vi "Add VIs and their Protperties to Tree.vi"(5 "Globals?":bool, 6 "File Extension Filters":string[](array[string]), 7 "Exclude vi.lib?":bool, 8 "error in":errorcluster, 10 "AppInst":refnum<vi>, 11 "Data Tree":refnum<vi>) -> (0 "error out":errorcluster)   [LabVIEW 2009]
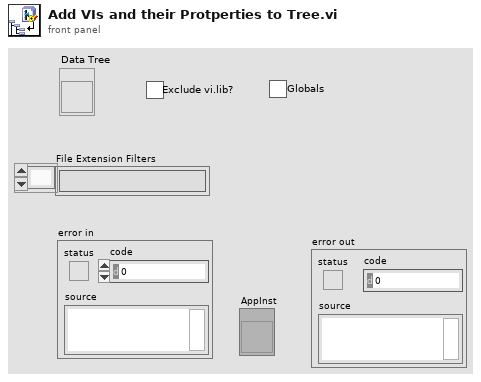
[diagram p1: front panel]
types:
  T1 = enum32{"invalid VI type", "Standard VI", "Control VI", "Global VI", "Polymorphic VI", "Configuration VI", "SubSystem", "Facade VI", "Method VI", "Statechart Diagram VI"}
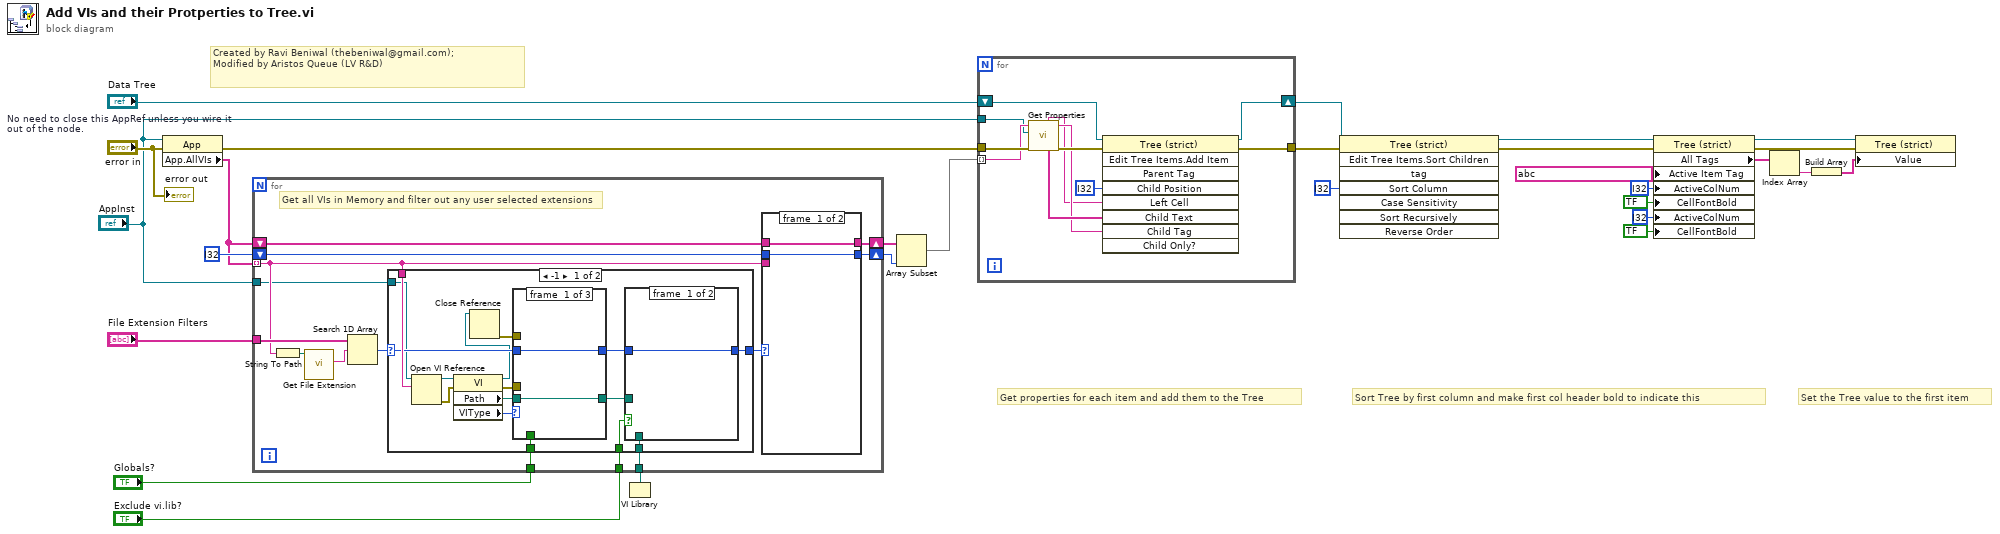
[diagram p0: block diagram]
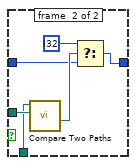
[diagram p2: hidden frame]
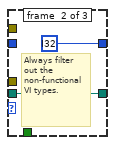
[diagram p3: hidden frame]
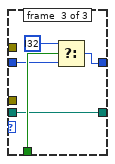
[diagram p4: hidden frame]
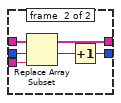
[diagram p6: hidden frame]
diagram:
  # "Sort Tree by first column and make first col header bold to indicate this"
  # "Created by Ravi Beniwal (thebeniwal@gmail.com);\nModified by Aristos Queue (LV R&D)"
  # "Set the Tree value to the first item"
  # "Get properties for each item and add them to the Tree"
  n1 = property on="No need to close this AppRef unless you wire it out of the node." class="App"(reference="AppInst", error in="error in") -> (error out=w5:errorcluster, "App.AllVIs"=w22:string[])  [unwired: 1 out]
  n2 = VI Library() -> (path=w2:path)
  n3 = for {
    tunnel: w22 -> [w33] mode=indexing
    tunnel: "File Extension Filters" -> [w41]
    shift-right: [w38] -> w24
    shift-left: w22 -> [w39]
    shift-right: [w36] -> w23
    shift-left: i32 ? -> [w37]
    tunnel: "Globals?" -> [w32]
    tunnel: "Exclude vi.lib?" -> [w31]
    tunnel: w2 -> [w30]
    tunnel: "AppInst" -> [w29]
    # "Get all VIs in Memory and filter out any user selected extensions"
    n4 = String To Path(string=w33) -> (path=w42:path)
    n5 = call <vilib>:"Get File Extension.vi"("file"=w42) -> ("lowercase file extension"=w40:string)  [unwired: 7 in, 3 out]
    n6 = Search 1D Array(1D array=w41, element=w40) -> (index of element=w35:i32)  [unwired: 1 in]
    n7 = case shown="-1" w35 {
      selector: w35 -> [w55 w75]
      tunnel: [w48 w75] -> w34
      tunnel: w33 -> [w58 _]
      tunnel: w32 -> [w53 _]
      tunnel: w31 -> [w52 _]
      tunnel: w30 -> [w50 _]
      tunnel: w29 -> [w43 _]
      frame #0 {
        n8 = Open VI Reference(application reference (local)=w43, vi path=w58) -> (vi reference=w57:refnum<vi>, error out=w46:errorcluster)  [unwired: 4 in]
        n9 = property class="VI"(reference=w57, error in=w46) -> (reference out=w47:refnum<vi>, error out=w45:errorcluster, "Path"=w54:path, "VIType"=w56:T1)
        n10 = Close Reference(reference=w47) -> (error out=w44:errorcluster)  [unwired: 1 in]
        n11 = case shown="\"Polymorphic VI\", \"Configuration VI\"" w56 {
          tunnel: w55 -> [w67 _ w73]
          tunnel: [w67 i32 ? ("index of element") w72] -> w49
          tunnel: w54 -> [w66 w68 w70]
          tunnel: w53 -> [_ _ w74]
          tunnel: [w66 w68 w70] -> w51
          tunnel: w45 -> [_ _ _]
          tunnel: w44 -> [_ _ _]
          frame #0 {
          }
          frame #1 {
            # "Always filter out the non-functional VI types."
          }
          frame #2 {
            n12 = Select(t=i32 ?, s=w74, f=w73) -> (s? t:f=w72:i32)
          }
        }
        n13 = case shown="True" w52 {
          tunnel: w51 -> [_ w65]
          tunnel: w50 -> [_ w64]
          tunnel: w49 -> [w59 w62]
          tunnel: [w59 w60] -> w48
          frame #0 {
          }
          frame #1 {
            n14 = call <vilib>:"Compare Two Paths.vi"("Path 2"=w65, "Path 1"=w64) -> ("Path 2 Relative to Path 1?"=w63:bool)  [unwired: 6 in, 3 out]
            n15 = Select(t=i32 ?, s=w63, f=w62) -> (s? t:f=w60:i32)
          }
        }
      }
      frame #1 {
      }
    }
    n16 = case shown="-1" w34 {
      tunnel: w39 -> [w77 w82]
      tunnel: [w77 w81] -> w38
      tunnel: w33 -> [_ w80]
      tunnel: w37 -> [w76 w79]
      tunnel: [w76 w78] -> w36
      frame #0 {
      }
      frame #1 {
        n17 = Replace Array Subset(array=w82, new element=w80, index=w79) -> (w81:string[])
        n18 = Increment(x=w79) -> (x+1=w78:i32)
      }
    }
  }
  n19 = Array Subset(array=w24, length=w23) -> (w21:string[])  [unwired: 1 in]
  n20 = for {
    tunnel: w21 -> [w86] mode=indexing
    tunnel: w5 -> [w89]
    tunnel: [w88] -> w18
    shift-right: [w87] -> w15
    shift-left: "Data Tree" -> [w92]
    tunnel: "AppInst" -> [w83]
    n21 = call "Get Properties.vi"("error in"=w89, "AppInst"=w83, "VI Name"=w86) -> ("error out"=w90:errorcluster, "Full Name Out"=w85:string, "VI Properties"=w91:string[], "File Name Out"=w84:string)  [unwired: 3 in, 2 out]
    n22 = invoke on="Invoke Node" class="Tree (strict)" method="Edit Tree Items.Add Item"(reference=w92, error in=w90, "Child Position"=i32 ?, "Left Cell"=w84, "Child Text"=w91, "Child Tag"=w85) -> (reference out=w87:refnum<vi>, error out=w88:errorcluster)  [unwired: 3 in, 7 out]
  }
  n23 = invoke on="Invoke Node" class="Tree (strict)" method="Edit Tree Items.Sort Children"(reference=w15, error in=w18, "Sort Column"=i32 ?) -> (reference out=w16:refnum<vi>, error out=w17:errorcluster)  [unwired: 5 in, 6 out]
  n24 = property class="Tree (strict)"(reference=w16, error in=w17, "Active Item Tag"=string ? ("Active Item:Tag"), "ActiveColNum"=i32 ? ("Active Cell:Active Column Number"), "CellFontBold"=bool ? ("Active Cell:Cell Font:Bold"), "ActiveColNum"=i32 ? ("Active Cell:Active Column Number"), "CellFontBold"=bool ? ("Active Cell:Cell Font:Bold")) -> (reference out=w12:refnum<vi>, error out=w13:errorcluster, "All Tags"=w14:string[])
  n25 = Index Array(array=w14) -> (element=w11:string)  [unwired: 1 in]
  n26 = Build Array(w11) -> (w20:string[])
  n27 = property class="Tree (strict)"(reference=w12, error in=w13, "Value"=w20) -> ()  [unwired: 2 out]
  "error out" <- "error in"
